vi "Exclusion.vi"(1 "PulseyCentre":i32=41801 min=0 max=1000000 step=1000, 3 "Paramètre Instrumentaux Avant":string[][](table)=[["Simon", "8", "23", "3450", "1", "", "", "", "", "", "", ""], ["Cpapir", "30", "34", "3530", "1", "", "", "", "", "", "", ""], ["Spectro", "2", "18", "3430", "1", "", "", "", "", "", "", ""], ["EEV F/8", "15", "30", "3840", "1", "", "", "", "", "", "", ""], ["Panoramix+EEV", "22", "30", "4500", "1", "", "", "", "", "", "", ""], ["FantOMM", "15", "26", "4300", "1", "", "", "", "", "", "", ""], ["EspiOMM", "12", "25", "3375", "1", "", "", "", "", "", "", ""], ["La Poune (F/15)", "1", "18", "4100", "1", "", "", "", "", "", "", ""], ["Panoramix2", "48", "43", "0", "1", "", "", "", "", "", "", ""]] caption="Paramètre Instrumentaux", 4 "Instrument":u16(ring) items=["Simon", "Cpapir", "Spectro", "EEV F/8", "Panoramix+EEV", "FantOMM", "EspiOMM", "La Poune (F/15)", "Panoramix2", "Simon+PolBOMM"], 5 "PulsexCentre":i32=641444 min=0 max=1000000 step=1000, 6 "CentreTel Y":i32=70736 min=0 max=1000000 step=1000, 7 "CentreTel X":i32=647041 min=0 max=1000000 step=1000, 8 "Range":dbl=52.8 format="%.2f", 9 "Rot(rad)":dbl=3.6441621315637374 step=0.1 format="%.2f", 10 "acrmin/pulse":dbl=5.28e-05 format="%.4e") -> (0 "Paramètre Instrumentaux Après":string[][](table)=[["Simon", "8", "23", "3450", "1", "", "", "", "", "", "", ""], ["Cpapir", "30", "34", "3530", "1", "", "", "", "", "", "", ""], ["Spectro", "2", "18", "3430", "1", "", "", "", "", "", "", ""], ["EEV F/8", "15", "30", "3840", "1", "", "", "", "", "", "", ""], ["Panoramix+EEV", "22", "30", "4500", "1", "", "", "", "", "", "", ""], ["FantOMM", "15", "26", "4300", "1", "", "", "", "", "", "", ""], ["EspiOMM", "12", "25", "3375", "1", "", "", "", "", "", "", ""], ["La Poune (F/15)", "1", "18", "4100", "1", "", "", "", "", "", "", ""], ["Panoramix2", "48", "43", "0", "1", "", "", "", "", "", "", ""]] caption="Paramètre Instrumentaux")   [LabVIEW 2010]
uses:
  Globals.vi
panel:
  in  "Terminé":bool
  in  "copypos":bool
  in  "Accept":bool
  out "Position actuelle":string
  out "TableXYPos":cluster{dbl[], dbl[]}[](graph)=[{[4.0, 4.0], [4.0, -4.0]}, {[4.0, -4.0], [-4.0, -4.0]}, {[-4.0, -4.0], [-4.0, 4.0]}, {[-4.0, 4.0], [4.0, 4.0]}, {array[201 elements], array[201 elements]}, {[-13.478014600952905, 16.74193585836962], [-18.637143622789957, 15.770465551601118]}, {[-54.16002143357691, -12.031862295047375], [20.010258640653248, -16.99059415490716]}, {[-12.031862295047375, 24.968990500513033], [-16.99059415490716, 25.137564983622372]}, {[24.968990500513033, -17.1591686380165], [25.137564983622372, 62.13841777918278]}, {[-54.16002143357691, -17.1591686380165], [20.010258640653248, 62.13841777918278]}]
  in  "2e couple":string
  in  "1er couple":string
  in  "ANNULER":bool
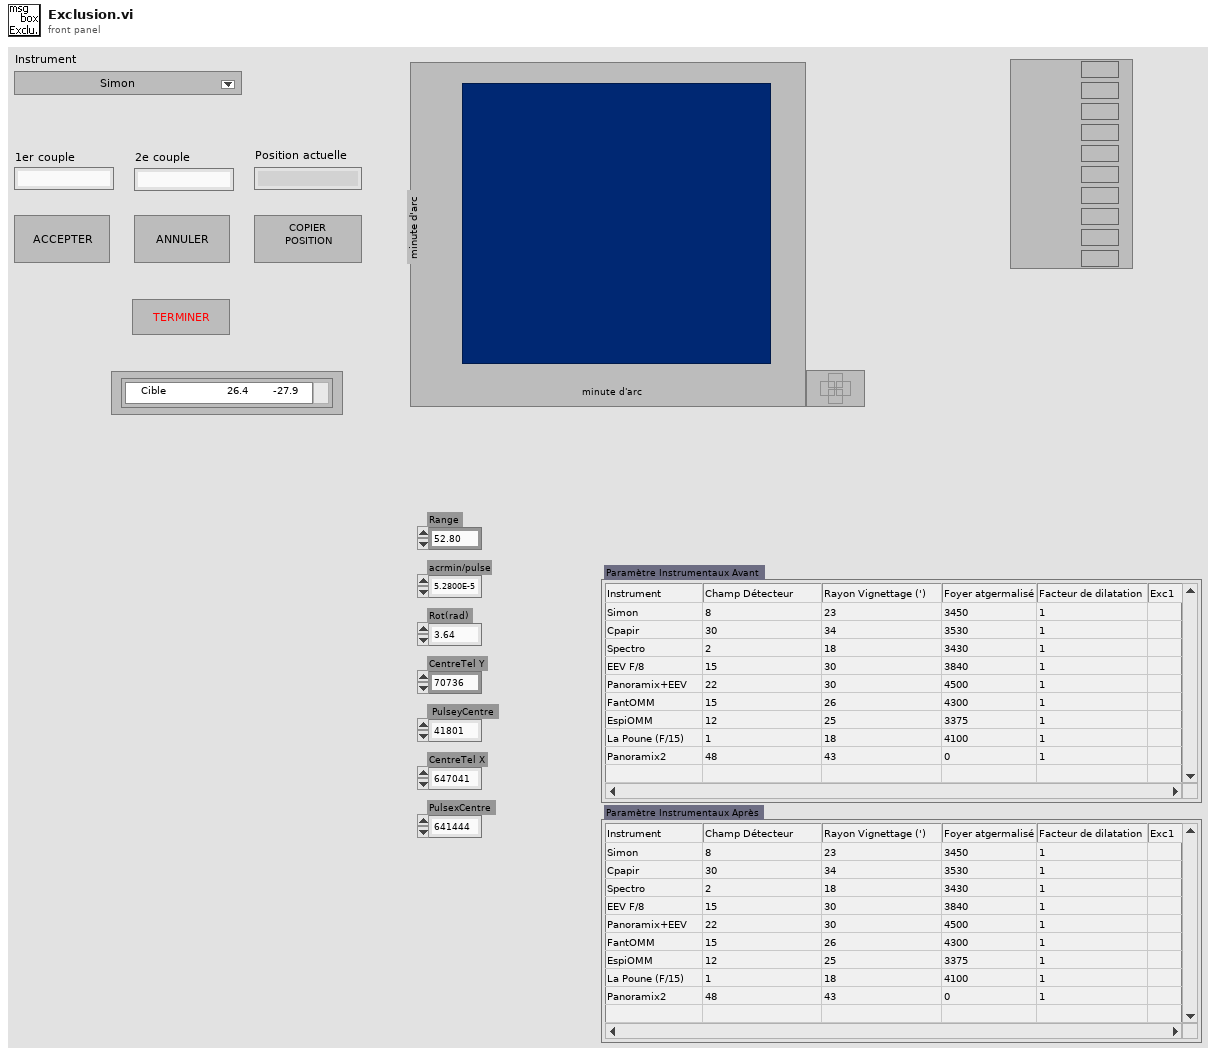
[diagram p1: front panel]
types:
  T1 = enum16{"Left Button", "Center Button", "Right Button", "Window Close"}
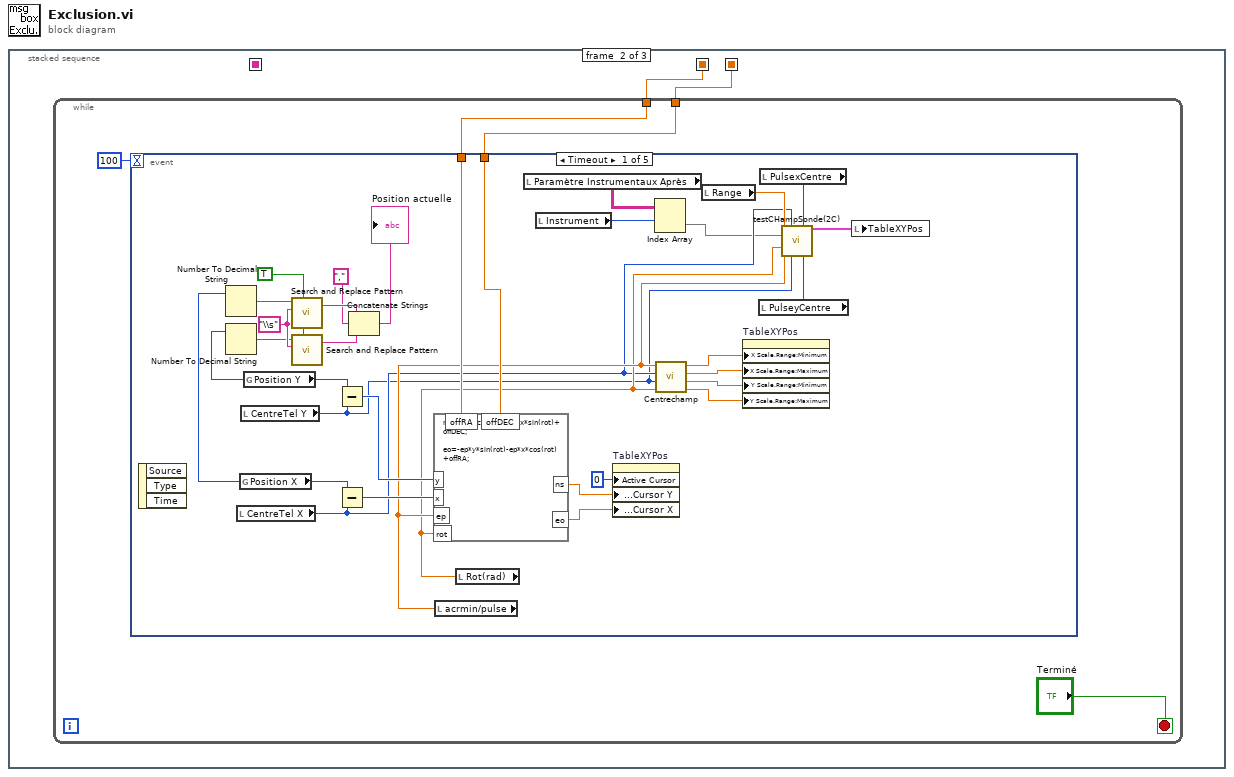
[diagram p0: block diagram]
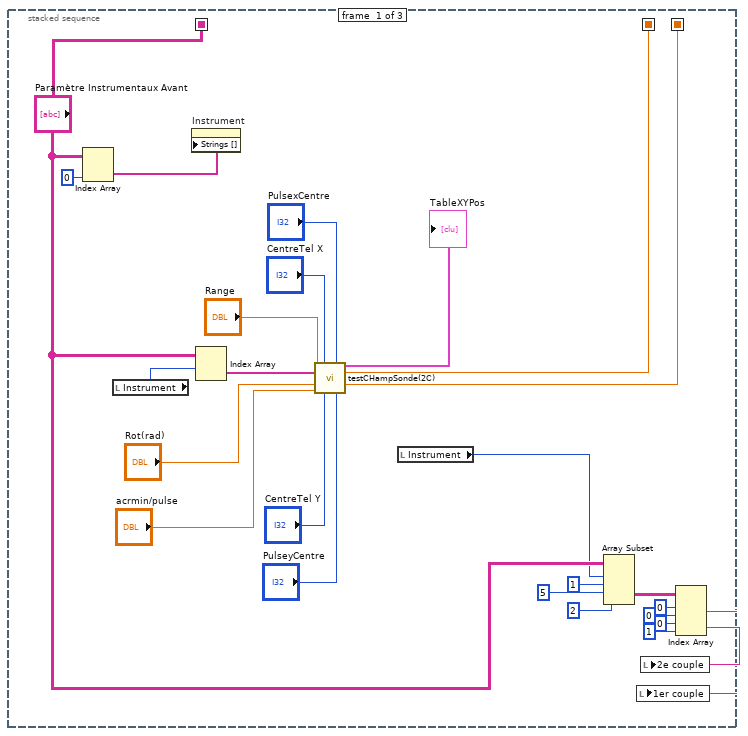
[diagram p2: hidden frame]
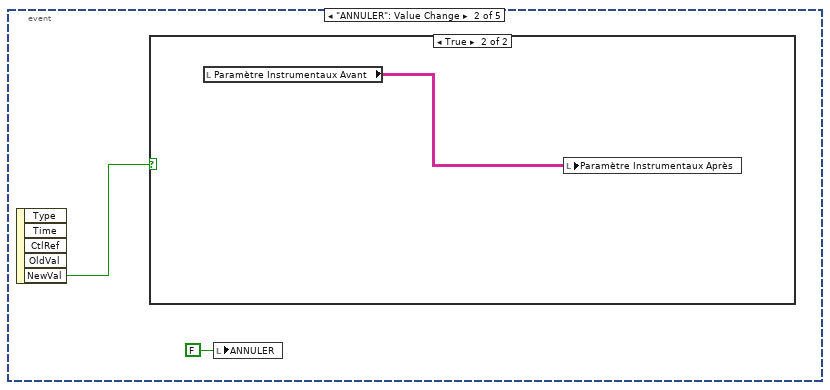
[diagram p3: hidden frame]
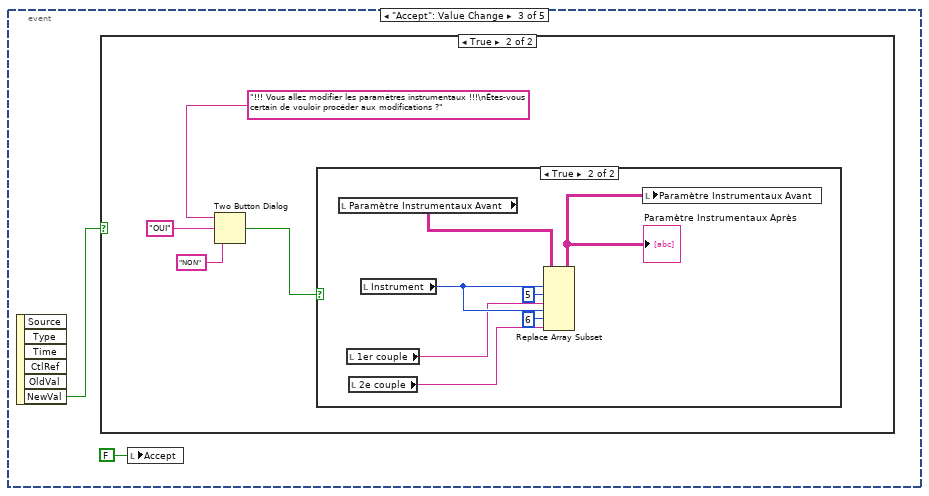
[diagram p5: hidden frame]
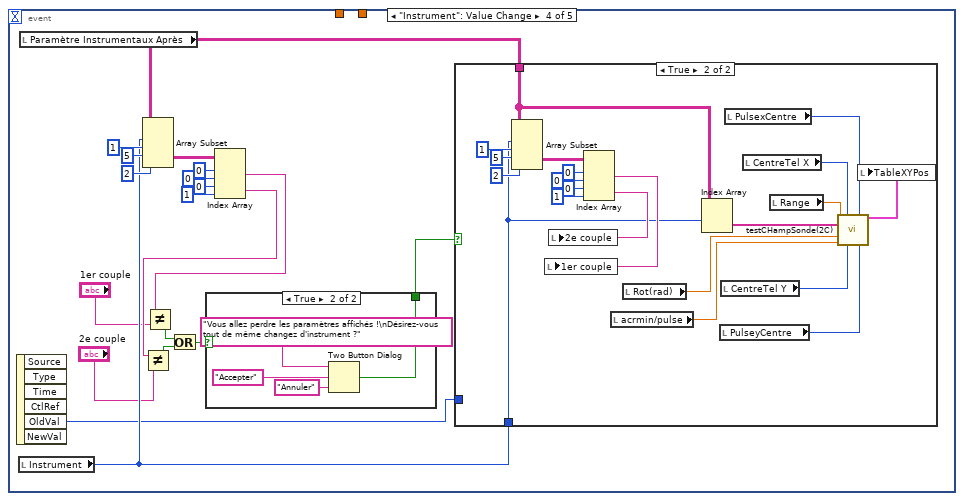
[diagram p8: hidden frame]
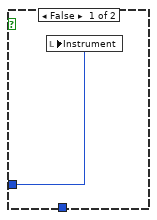
[diagram p10: hidden frame]
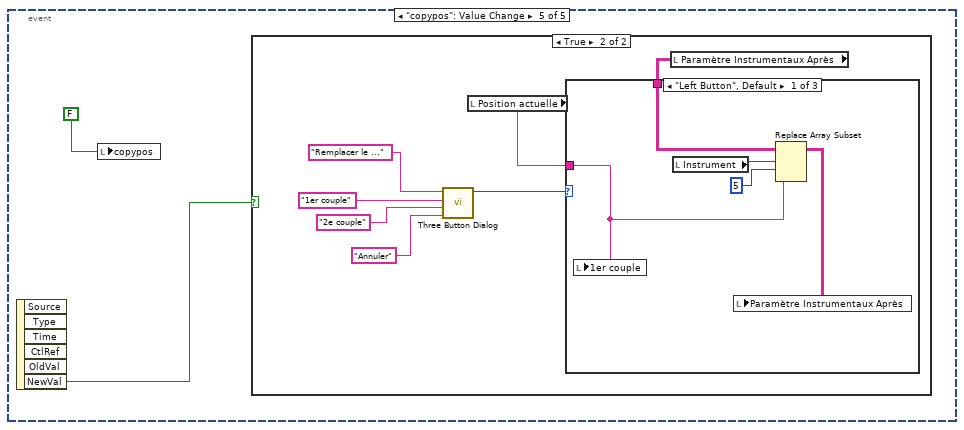
[diagram p11: hidden frame]
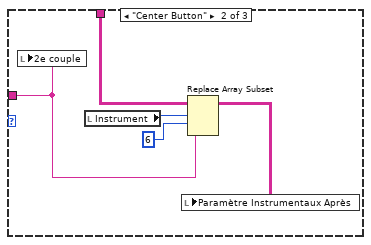
[diagram p13: hidden frame]
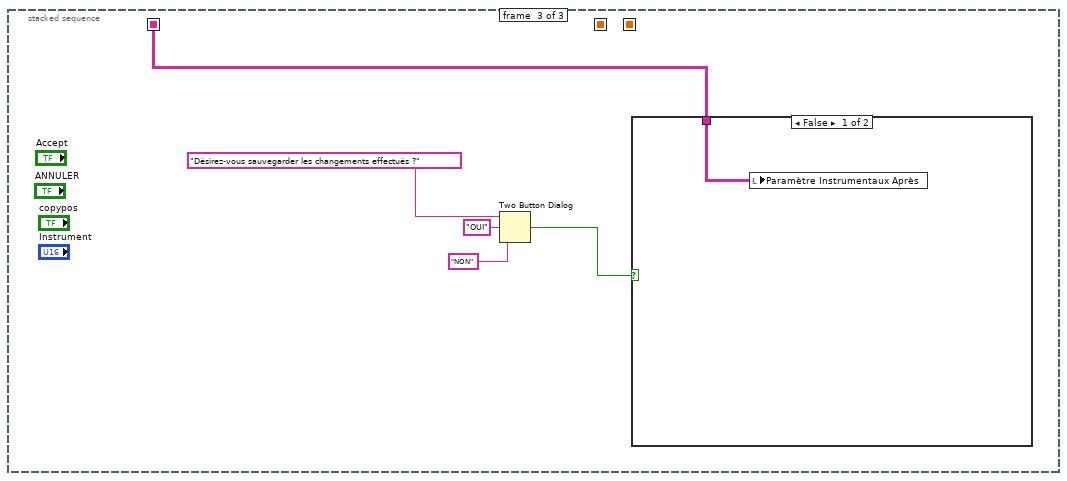
[diagram p15: hidden frame]
diagram:
  n1 = stacked-sequence {
    seq-local: [w16 _ _] -> [_ w28 _]
    seq-local: [w15 _ _] -> [_ w27 _]
    seq-local: ["Paramètre Instrumentaux Avant" _ _] -> [_ _ w146]
    frame #0 {
      n2 = Index Array(array="Paramètre Instrumentaux Avant", index (col)=0 ("disabled index (col)")) -> (element=w26:string[])  [unwired: 1 in]
      n3 = local read "Instrument"() -> (w1:u16)
      n4 = property on="Instrument" class="Ring (strict)"("Strings []"=w26) -> ()  [unwired: 2 in, 2 out]
      n5 = Index Array(array="Paramètre Instrumentaux Avant", index (row)=w1) -> (element=w2:string[])  [unwired: 1 in]
      n6 = call "testCHampSonde(2C).vi"("Range"="Range", "CentreTel X"="CentreTel X", "PulsexCentre"="PulsexCentre", "ParametresInstrumentaux"=w2, "Rot(rad)"="Rot(rad)", "acrmin/pulse"="acrmin/pulse", "CentreTel Y"="CentreTel Y", "PulseyCentre"="PulseyCentre") -> ("Champ"=→"TableXYPos":cluster{dbl[], dbl[]}[], "offRA"=w16:dbl, "offDEC"=w15:dbl)  [unwired: 4 in, 1 out]
      n7 = local read "Instrument"() -> (w3:u16)
      n8 = Array Subset(array="Paramètre Instrumentaux Avant", index (row)=w3, length (row)=1 ("length"), index (col)=5 ("index"), length (col)=2 ("length")) -> (w11:string[][])
      n9 = Index Array(array=w11, index (row) #1=0 ("index (row)"), index (col) #1=0 ("disabled index (col)"), index (row) #2=0 ("index (row)"), index (col) #2=1 ("disabled index (col)")) -> (element #1=w8:string, element #2=w7:string)
      n10 = local write "1er couple"(w8) -> ()
      n11 = local write "2e couple"(w7) -> ()
    }
    frame #1 {
      n12 = while {
        tunnel: w28 -> [w32]
        tunnel: w27 -> [w31]
        stop <- "Terminé" stop-if-true
        n13 = event shown="[0] Timeout" {
          selector: _ -> [_ _ _ _ _]
          dyn-events: _ -> [_ _ _ _ _]
          timeout: 100 -> [_ _ _ _ _]
          tunnel: w32 -> [w59 _ _ _ _]
          tunnel: w31 -> [w58 _ _ _ _]
          event Timeout {
            w55 = TRUE ("replace all? (F)")
            w57 = "\\s" ("regular expression (\"\")")
            n14 = event-data() -> ()  [unwired: 1 in, 3 out]
            n15 = local read "CentreTel X"() -> (w45:i32)
            n16 = global read "Globals.vi" "Position X"() -> (w38:i32)
            n17 = Number To Decimal String(number=w38) -> (decimal integer string=w40:string)  [unwired: 1 in]
            n18 = local read "CentreTel Y"() -> (w44:i32)
            n19 = global read "Globals.vi" "Position Y"() -> (w39:i32)
            n20 = Number To Decimal String(number=w39) -> (decimal integer string=w41:string)  [unwired: 1 in]
            n21 = call <vilib>:"Search and Replace Pattern.vi"("string"=w40, "regular expression (\"\")"=w57, "replace all? (F)"=w55) -> ("result string"=w56:string)  [unwired: 2 in, 1 out]
            n22 = call <vilib>:"Search and Replace Pattern.vi"("string"=w41, "regular expression (\"\")"=w57, "replace all? (F)"=w55) -> ("result string"=w36:string)  [unwired: 2 in, 1 out]
            n23 = Subtract(x=w39, y=w44) -> (x-y=w63:i32)
            n24 = Subtract(x=w38, y=w45) -> (x-y=w64:i32)
            n25 = Concatenate Strings(w56, "," ("regular expression (\"\")"), w36) -> (→"Position actuelle":string)
            n26 = local read "acrmin/pulse"() -> (w48:dbl)
            n27 = local read "Rot(rad)"() -> (w47:dbl)
            n28 = formula code="ns=ep*y*cos(rot)-ep*x*sin(rot)+offDEC;\n\neo=-ep*y*sin(rot)-ep*x*cos(rot)+offRA;"("y"=w63, "x"=w64, "ep"=w48, "rot"=w47, "offRA"=w59, "offDEC"=w58) -> ("eo"=w61:dbl, "ns"=w62:dbl)
            n29 = local read "Paramètre Instrumentaux Après"() -> (w35:string[][])
            n30 = local read "Instrument"() -> (w34:u16)
            n31 = property on="TableXYPos" class="XYGraph (strict)"("Active Cursor"=u32 0, "Cursor.Cursor Position:Cursor Y"=w62, "Cursor.Cursor Position:Cursor X"=w61) -> ()  [unwired: 2 in, 2 out]
            n32 = Index Array(array=w35, index (row)=w34) -> (element=w33:string[])  [unwired: 1 in]
            n33 = call "Centrechamp.vi"("Rot(rad)"=w47, "CentreTelY"=w44, "CentreTelX"=w45, "arcmin/pulse"=w48) -> ("Max Y"=w53:dbl, "Min Y"=w52:dbl, "Max X"=w51:dbl, "Min X"=w50:dbl)
            n34 = local read "Range"() -> (w46:dbl)
            n35 = property on="TableXYPos" class="XYGraph (strict)"("X Scale.Range:Minimum"=w50, "X Scale.Range:Maximum"=w51, "Y Scale.Range:Minimum"=w52, "Y Scale.Range:Maximum"=w53) -> ()  [unwired: 2 in, 2 out]
            n36 = local read "PulseyCentre"() -> (w42:i32)
            n37 = local read "PulsexCentre"() -> (w43:i32)
            n38 = call "testCHampSonde(2C).vi"("Range"=w46, "CentreTel X"=w45, "PulsexCentre"=w43, "ParametresInstrumentaux"=w33, "Rot(rad)"=w47, "acrmin/pulse"=w48, "CentreTel Y"=w44, "PulseyCentre"=w42) -> ("Champ"=w49:cluster{dbl[], dbl[]}[])  [unwired: 4 in, 3 out]
            n39 = local write "TableXYPos"(w49) -> ()
          }
          event "ANNULER": Value Change {
            n40 = event-data() -> ("NewVal"=w66:bool)  [unwired: 1 in, 4 out]
            n41 = case shown="True" w66 {
              frame False {
              }
              frame True {
                n42 = local read "Paramètre Instrumentaux Avant"() -> (w67:string[][])
                n43 = local write "Paramètre Instrumentaux Après"(w67) -> ()
              }
            }
            n44 = local write "ANNULER"(FALSE ("ANNULER")) -> ()
          }
          event "Accept": Value Change {
            n45 = event-data() -> ("NewVal"=w69:bool)  [unwired: 1 in, 5 out]
            n46 = case shown="True" w69 {
              frame False {
              }
              frame True {
                n47 = Two Button Dialog(message="!!! Vous allez modifier les paramètres instrumentaux !!!\nÊtes-vous certain de vouloir procéder aux modifications ?", 1:"NON" ("F button name (\"Cancel\")"), 2:"OUI" ("T button name (\"OK\")")) -> (T button?=w73:bool)
                n48 = case shown="True" w73 {
                  frame False {
                  }
                  frame True {
                    n49 = local read "Paramètre Instrumentaux Avant"() -> (w75:string[][])
                    n50 = local read "1er couple"() -> (w77:string)
                    n51 = local read "2e couple"() -> (w76:string)
                    n52 = local read "Instrument"() -> (w80:u16)
                    n53 = Replace Array Subset(array=w75, new element #1=w77, index (row) #1=w80, index (col) #1=5 ("disabled index (col)"), new element #2=w76, index (row) #2=w80, index (col) #2=6 ("disabled index (col)")) -> (w74:string[][])
                    "Paramètre Instrumentaux Après" <- w74
                    n54 = local write "Paramètre Instrumentaux Avant"(w74) -> ()
                  }
                }
              }
            }
            n55 = local write "Accept"(FALSE ("Accept")) -> ()
          }
          event "Instrument": Value Change {
            n56 = event-data() -> ("OldVal"=w81:u16)  [unwired: 1 in, 5 out]
            n57 = local read "Instrument"() -> (w92:u16)
            n58 = local read "Paramètre Instrumentaux Après"() -> (w91:string[][])
            n59 = Array Subset(array=w91, index (row)=w92, length (row)=1 ("length"), index (col)=5 ("index"), length (col)=2 ("length")) -> (w96:string[][])
            n60 = Index Array(array=w96, index (row) #1=0 ("index (row)"), index (col) #1=0 ("disabled index (col)"), index (row) #2=0 ("index (row)"), index (col) #2=1 ("disabled index (col)")) -> (element #1=w88:string, element #2=w87:string)
            n61 = Not Equal?(x=w87, y="2e couple") -> (x != y?=w90:bool)
            n62 = Not Equal?(x=w88, y="1er couple") -> (x != y?=w89:bool)
            n63 = Or(x=w89, y=w90) -> (x .or. y?=w83:bool)
            n64 = case shown="True" w83 {
              selector: w83 -> [w100 _]
              tunnel: [w100 w104] -> w84
              frame False {
              }
              frame True {
                n65 = Two Button Dialog(message="Vous allez perdre les paramètres affichés !\nDésirez-vous tout de même changez d'instrument ?", 1:"Annuler" ("F button name (\"Cancel\")"), 2:"Accepter" ("F button name (\"Cancel\")")) -> (T button?=w104:bool)
              }
            }
            n66 = case shown="True" w84 {
              tunnel: w91 -> [_ w108]
              tunnel: w92 -> [_ w106]
              tunnel: w81 -> [w105 _]
              frame False {
                n67 = local write "Instrument"(w105) -> ()
              }
              frame True {
                n68 = Array Subset(array=w108, index (row)=w106, length (row)=1 ("length"), index (col)=5 ("index"), length (col)=2 ("length")) -> (w118:string[][])
                n69 = Index Array(array=w118, index (row) #1=0 ("index (row)"), index (col) #1=0 ("disabled index (col)"), index (row) #2=0 ("index (row)"), index (col) #2=1 ("disabled index (col)")) -> (element #1=w115:string, element #2=w114:string)
                n70 = local write "1er couple"(w115) -> ()
                n71 = local write "2e couple"(w114) -> ()
                n72 = local read "acrmin/pulse"() -> (w109:dbl)
                n73 = local read "Rot(rad)"() -> (w110:dbl)
                n74 = Index Array(array=w108, index (row)=w106) -> (element=w107:string[])  [unwired: 1 in]
                n75 = local read "PulseyCentre"() -> (w125:i32)
                n76 = local read "CentreTel Y"() -> (w126:i32)
                n77 = local read "PulsexCentre"() -> (w123:i32)
                n78 = local read "CentreTel X"() -> (w124:i32)
                n79 = local read "Range"() -> (w111:dbl)
                n80 = call "testCHampSonde(2C).vi"("Range"=w111, "CentreTel X"=w124, "PulsexCentre"=w123, "ParametresInstrumentaux"=w107, "Rot(rad)"=w110, "acrmin/pulse"=w109, "CentreTel Y"=w126, "PulseyCentre"=w125) -> ("Champ"=w122:cluster{dbl[], dbl[]}[])  [unwired: 4 in, 3 out]
                n81 = local write "TableXYPos"(w122) -> ()
              }
            }
          }
          event "copypos": Value Change {
            n82 = event-data() -> ("NewVal"=w128:bool)  [unwired: 1 in, 5 out]
            n83 = local write "copypos"(FALSE) -> ()
            n84 = case shown="True" w128 {
              frame False {
              }
              frame True {
                n85 = call <vilib>:"Three Button Dialog.vi"("Right Button Text (\"Cancel\")"="Annuler" ("Right Button Text (\"Cancel\")"), "Center Button Text (\"No\")"="2e couple" ("F button name (\"Cancel\")"), "Left Button Text (\"Yes\")"="1er couple" ("F button name (\"Cancel\")"), "message"="Remplacer le ...") -> ("Which Button?"=w131:T1)  [unwired: 7 in]
                n86 = local read "Position actuelle"() -> (w130:string)
                n87 = local read "Paramètre Instrumentaux Après"() -> (w129:string[][])
                n88 = case shown="\"Left Button\", Default" w131 {
                  tunnel: w130 -> [w136 w142 _]
                  tunnel: w129 -> [w137 w145 _]
                  frame "Left Button", Default {
                    n89 = local write "1er couple"(w136) -> ()
                    n90 = local read "Instrument"() -> (w140:u16)
                    n91 = Replace Array Subset(array=w137, new element=w136, index (row)=w140, index (col)=5 ("disabled index (col)")) -> (w138:string[][])
                    n92 = local write "Paramètre Instrumentaux Après"(w138) -> ()
                  }
                  frame "Center Button" {
                    n93 = local write "2e couple"(w142) -> ()
                    n94 = local read "Instrument"() -> (w144:u16)
                    n95 = Replace Array Subset(array=w145, new element=w142, index (row)=w144, index (col)=6 ("disabled index (col)")) -> (w141:string[][])
                    n96 = local write "Paramètre Instrumentaux Après"(w141) -> ()
                  }
                  frame "Right Button" {
                  }
                }
              }
            }
          }
        }
      }
    }
    frame #2 {
      n97 = Two Button Dialog(message="Désirez-vous sauvegarder les changements effectués ?", 1:"NON" ("F button name (\"Cancel\")"), 2:"OUI" ("T button name (\"OK\")")) -> (T button?=w147:bool)
      n98 = case shown="False" w147 {
        tunnel: w146 -> [w151 _]
        frame False {
          n99 = local write "Paramètre Instrumentaux Après"(w151) -> ()
        }
        frame True {
        }
      }
    }
  }
